vi "Get Path.vi"(8 "error in (no error)":errorcluster, 11 "WebProjectPanel in":refnum<class "WebProjectPanel.lvclass">) -> (0 "error out":errorcluster, 2 "Path":path, 3 "WebProjectPanel out":refnum<class "WebProjectPanel.lvclass">)   [LabVIEW 2020, in "PicoG-Processor.lvlib" / "WebProjectPanel.lvclass"]
uses:
  WebProjectPanel.lvclass
  WebProjectPanel.lvclass/WebProjectPanel.ctl
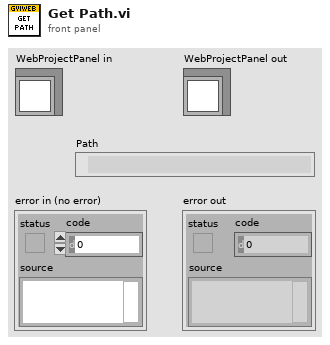
[diagram p1: front panel]
types:
  T1 = typedef "PicoG-Processor.lvlib/WebProjectPanel.lvclass/Ref Data.ctl" = cluster{"Last Update":dbl, "Path":path, "App Name":string, "Build Present":bool, "Deploy":refnum<user-event>}
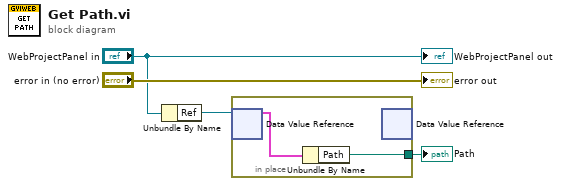
[diagram p0: block diagram]
diagram:
  n1 = Unbundle By Name("WebProjectPanel in") -> ("Ref"=w3:refnum<data-value>)
  n2 = in-place {
    in-place-border: [w5] -> w1
    n3 = in-place-dvr #1(w3) -> (w6:T1)  [unwired: 1 out]
    n4 = Unbundle By Name(w6) -> ("Path"=w5:path)
    n5 = in-place-dvr #1() -> ()  [unwired: 1 in, 2 out]
  }
  "Path" <- w1
  "error out" <- "error in (no error)"
  "WebProjectPanel out" <- "WebProjectPanel in"
